vi "Example NetworkQueue Client-Server.vi"() -> ()   [LabVIEW 2013]
uses:
  Connection/Connection.lvclass
  Connection.NetworkQueue/Connection.NetworkQueue.lvclass
panel:
  out "server connected":bool
  out "client connected":bool
  out "Comm OK":bool
  out "value":dbl
  out "listener error":errorcluster
  out "client session error":errorcluster
  out "server session error":errorcluster
  out "Bytes":u8[](array[numeric]) format="%08b"
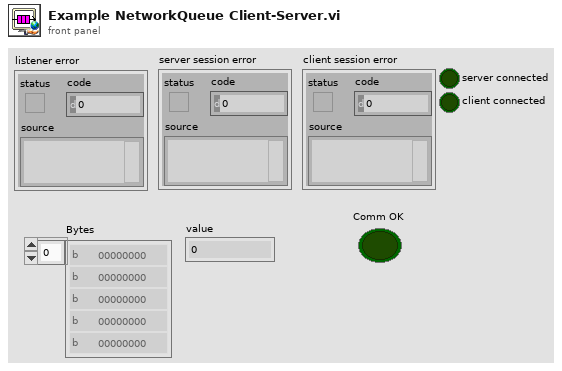
[diagram p1: front panel]
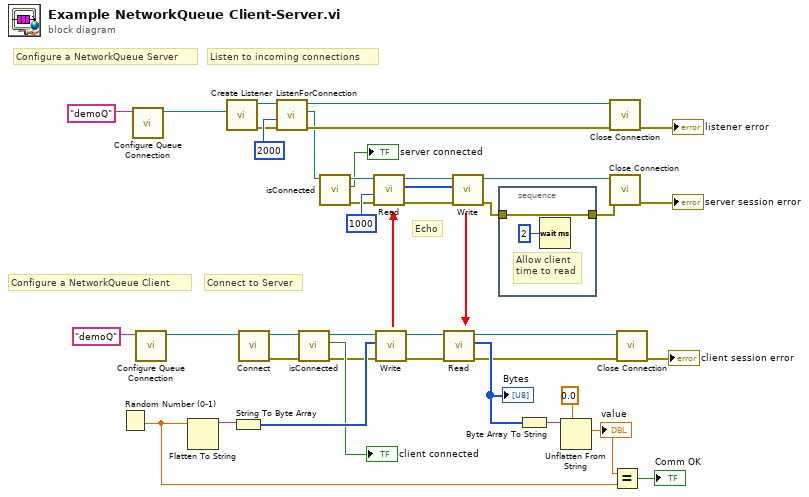
[diagram p0: block diagram]
diagram:
  # "Configure a NetworkQueue Client"
  # "Connect to Server"
  # "Echo"
  # "Listen to incoming connections"
  # "Configure a NetworkQueue Server"
  n1 = Random Number (0-1)() -> (number: 0 to 1=w17:dbl)
  n2 = call "Configure Queue Connection.vi"("Queue Name"="demoQ" ("address (localhost)")) -> ("Connection.LocalQueue"=w3:refnum<class "Connection.NetworkQueue.lvclass">)  [unwired: 9 in, 1 out]
  n3 = call "Configure Queue Connection.vi"("Queue Name"="demoQ" ("address (localhost)")) -> ("Connection.LocalQueue"=w1:refnum<class "Connection.NetworkQueue.lvclass">)  [unwired: 9 in, 1 out]
  n4 = Flatten To String(anything=w17) -> (data string=w28:string)  [unwired: 3 in, 2 out]
  n5 = call "Create Listener.vi"("Connection Configuration"=w3) -> ("error out"=w37:errorcluster, "Listener"=w40:refnum<class "Connection.lvclass">)  [unwired: 9 in]
  n6 = String To Byte Array(string=w28) -> (unsigned byte array=w27:u8[])
  n7 = call "Connect.vi"("Connection in"=w1) -> ("error out"=w12:errorcluster, "Connection out"=w10:refnum<class "Connection.NetworkQueue.lvclass">)  [unwired: 9 in]
  n8 = call "ListenForConnection.vi"("error in (no error)"=w37, "timeout (2000 ms)"=2000 ("bytes to read (100)"), "Listener"=w40) -> ("error out"=w22:errorcluster, "Connection"=w8:refnum<class "Connection.lvclass">, "Listener out"=w38:refnum<class "Connection.lvclass">)  [unwired: 5 in, 1 out]
  n9 = call "isConnected.vi"("error in (no error)"=w12, "Connection in"=w10) -> ("error out"=w11:errorcluster, "connected"=→"client connected":bool, "Connection out"=w9:refnum<class "Connection.NetworkQueue.lvclass">)  [unwired: 7 in]
  n10 = call "isConnected.vi"("Connection in"=w8) -> ("error out"=w6:errorcluster, "connected"=→"server connected":bool, "Connection out"=w7:refnum<class "Connection.lvclass">)  [unwired: 8 in]
  n11 = call "Read.vi"("error in (no error)"=w6, "timeout (2000 ms)"=1000 ("bytes to read (100)"), "TCPConnection in"=w7) -> ("error out"=w32:errorcluster, "Bytes"=w34:u8[], "TCPConnection out"=w35:refnum<class "Connection.lvclass">)  [unwired: 4 in, 2 out]
  n12 = call "Write.vi"("error in (no error)"=w11, "Bytes"=w27, "Connection in"=w9) -> ("error out"=w31:errorcluster, "Connection"=w33:refnum<class "Connection.NetworkQueue.lvclass">)  [unwired: 7 in]
  n13 = call "Read.vi"("error in (no error)"=w31, "TCPConnection in"=w33) -> ("error out"=w20:errorcluster, "Bytes"=w26:u8[], "TCPConnection out"=w19:refnum<class "Connection.NetworkQueue.lvclass">)  [unwired: 5 in, 2 out]
  "Bytes" <- w26
  n14 = call "Write.vi"("error in (no error)"=w32, "Bytes"=w34, "Connection in"=w35) -> ("error out"=w15:errorcluster, "Connection"=w29:refnum<class "Connection.lvclass">)  [unwired: 7 in]
  n15 = stacked-sequence {
    tunnel: w15 -> [w41]
    tunnel: [w41] -> w14
    frame #0 {
      # "Allow client\ntime to read"
      n16 = Wait (ms)(milliseconds to wait=u32 2) -> ()  [unwired: 1 out]
    }
  }
  n17 = Byte Array To String(unsigned byte array=w26) -> (string=w25:string)
  n18 = Unflatten From String(type=0.0, binary string=w25) -> (value=w18:dbl)  [unwired: 3 in, 2 out]
  "value" <- w18
  n19 = call "Close Connection.vi"("error in (no error)"=w22, "Connection in"=w38) -> ("error out"=→"listener error":errorcluster)  [unwired: 8 in, 1 out]
  n20 = call "Close Connection.vi"("error in (no error)"=w14, "Connection in"=w29) -> ("error out"=→"server session error":errorcluster)  [unwired: 8 in, 1 out]
  n21 = Equal?(x=w18, y=w17) -> (x = y?=→"Comm OK":bool)
  n22 = call "Close Connection.vi"("error in (no error)"=w20, "Connection in"=w19) -> ("error out"=→"client session error":errorcluster)  [unwired: 8 in, 1 out]
